vi "Mcp2210 Get Usb Key Params.vi"(0 "handle":i32, 11 "error in (no error)":errorcluster) -> (4 "handle out":i32, 6 "USB Status":T1 {"PID" format="%x"; "VID" format="%x"}, 15 "error out":errorcluster)   [LabVIEW 2015, in "mcp2210.lvlib"]
doc: "Provides the USB key configuration attributes: VID, PID and power settings.\nIn case of successful execution, the function returns 0 (M_E_SUCCESS) and updates the reference\nparameters with the settings values. In case of failure, negative error code is returned.\nParameters:\nInputs:\n- IntPtr handle - USB device handle. Cannot be NULL.\nOutputs:\n- unsigned short %pvid - device VID\n- unsigned short %ppid - device PID\n- unsigned char %ppwrSrc - device power source, according to USB 2.0 specs, chapter 9:\n- bit 7 = Host-Powered: 1=yes.\nThis bit is reserved and must be set to 1 for historical\nreasons.\n- bit 6 = Self-Powered: 1=yes; 0=no.\n- bits 5..0 = 0.\n- unsigned char %prmtWkup - device is remote wake-up capable: 1=yes; 0=no.\n- unsigned short %pcurrentLd - Maximum current consumption from the USB Host, expressed in mA.\nThe value is a multiple of 2, ranging from 2mA to 510mA.\nReturns:\n- 0 for success: M_E_SUCCESS\n- negative error code: M_E_ERR_NULL, M_E_ERR_INVALID_HANDLE_VALUE\nM_E_ERR_HID_TIMEOUT, M_E_ERR_HID_RW_FILEIO, M_E_ERR_UNKOWN_ERROR\nM_E_ERR_CMD_ECHO, M_E_ERR_CMD_FAILED\n\nMCP2210_DLL_UM_API int __stdcall Mcp2210_GetUsbKeyParams(void *handle, unsigned short *pvid, unsigned short *ppid,\n unsigned char *ppwrSrc, unsigned char *prmtWkup, unsigned short *pcurrentLd);"
uses:
  <userlib>/mcp2210/mcp2210.lvlib
  <userlib>/mcp2210/mcp2210_dll_um_x86.dll
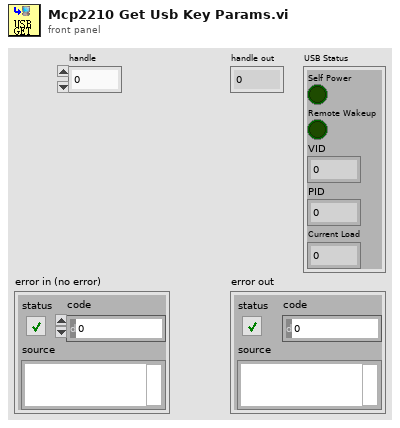
[diagram p1: front panel]
types:
  T1 = cluster{"Self Power":bool, "Remote Wakeup":bool, "VID":u16, "PID":u16, "Current Load":u16}
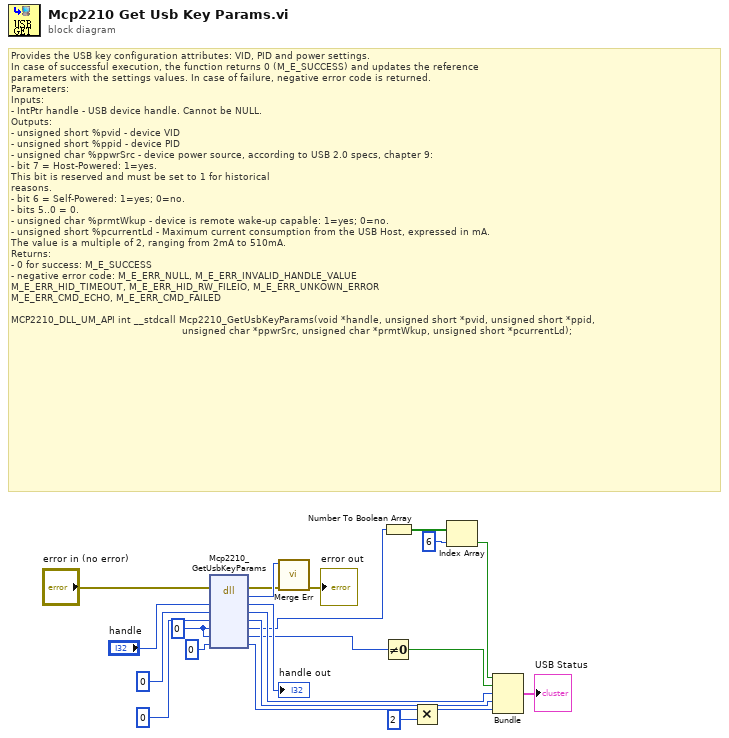
[diagram p0: block diagram]
diagram:
  w2 = u8 0 ("ppwrSrc")
  # "Provides the USB key configuration attributes: VID, PID and power settings.\nIn case of successful execution, the function returns 0 (M_E_SUCCESS) and updates the reference\nparameters with the settings values. In case of failure, negative error code is returned.\nParameters:\nInputs:\n- IntPtr handle - USB device handle. Cannot be NULL.\nOutputs:\n- unsigned short %pvid - device VID\n- unsigned short %ppid - device PID\n- unsigned char %ppwrSrc - device power source, according to USB 2.0 specs, chapter 9:\n- bit 7 = Host-Powered: 1=yes.\nThis bit is reserved and must be set to 1 for historical\nreasons.\n- bit 6 = Self-Powered: 1=yes; 0=no.\n- bits 5..0 = 0.\n- unsigned char %prmtWkup - device is remote wake-up capable: 1=yes; 0=no.\n- unsigned short %pcurrentLd - Maximum current consumption from the USB Host, expressed in mA.\nThe value is a multiple of 2, ranging from 2mA to 510mA.\nReturns:\n- 0 for success: M_E_SUCCESS\n- negative error code: M_E_ERR_NULL, M_E_ERR_INVALID_HANDLE_VALUE\nM_E_ERR_HID_TIMEOUT, M_E_ERR_HID_RW_FILEIO, M_E_ERR_UNKOWN_ERROR\nM_E_ERR_CMD_ECHO, M_E_ERR_CMD_FAILED\n\nMCP2210_DLL_UM_API int __stdcall Mcp2210_GetUsbKeyParams(void *handle, unsigned short *pvid, unsigned short *ppid,\n                                                         unsigned char *ppwrSrc, unsigned char *prmtWkup, unsigned short *pcurrentLd);"
  n1 = dll-call lib="D:/LabVIEW 2015/user.lib/mcp2210/mcp2210_dll_um_x86.*" fn="Mcp2210_GetUsbKeyParams"(error in="error in (no error)", "handle"="handle", "pvid"=u16 0, "ppid"=u16 0, "ppwrSrc"=w2, "prmtWkup"=w2, "pcurrentLd"=u16 0) -> (error out=w14:errorcluster, "return type"=w15:i32, "handle"=→"handle out":u32, "pvid"=w10:u16, "ppid"=w9:u16, "ppwrSrc"=w3:u8, "prmtWkup"=w1:u8, "pcurrentLd"=w8:u16)  [unwired: 2 in, 1 out]
  n2 = call <userlib>:"Merge Err.vi"("error in (no error)"=w14, "return type"=w15) -> ("error out"=→"error out":errorcluster)  [unwired: 9 in]
  n3 = Not Equal To 0?(x=w1) -> (x != 0?=w11:bool)
  n4 = Number To Boolean Array(number=w3) -> (Boolean array=w17:bool[])
  n5 = Multiply(x=w8, y=u16 2) -> (x*y=w5:u16)
  n6 = Index Array(array=w17, index=6) -> (element=w12:bool)
  n7 = Bundle(w12, w11, "pvid"=w10, "ppid"=w9, w5) -> (→"USB Status":cluster{bool, bool, "pvid":u16, "ppid":u16, u16})  [unwired: 1 in]
